vi "Wheel_Control_POS.vi"(9 "CW is Up":bool=TRUE, 10 "AIDeviceRef":T1={"DevStatus"={"status"=FALSE, "code"=0, "source"=""}, "Analog Channel"=enum."AI 1"}, 11 "Wheel DevRef In":T3) -> ()   [LabVIEW 2015, in "Wheel.lvlib"]
doc: "Help by FRC 836 - The RoboBees\n\nThis VI sets the shooter wheel postion using a PID control VI with parameters set by\nthe tbh (Take Back Half) control VI."
uses:
  <userlib>/836-Library/Motion_Control/Shooter_Wheel/Wheel.lvlib
  <userlib>/836-Library/Motion_Control/Shooter_Wheel/WheelControl.ctl
  <userlib>/836-Library/Motion_Control/Shooter_Wheel/Config.ctl
  <userlib>/836-Library/Motion_Control/Shooter_Wheel/Data.ctl
  <vilib>/Rock Robotics/WPI/MotorControl/WPI_MotorControlDeviceRef.ctl
  <vilib>/Rock Robotics/WPI/MotorControl/WPI_MotorControlType.ctl
  <vilib>/Rock Robotics/SystemInterfaces/DIO/FPGA_DIOPWMChannel.ctl
  <vilib>/Rock Robotics/WPI/PWM/WPI_PWMDeadband.ctl
  <vilib>/Rock Robotics/WPI/CAN/Jaguar/SubVIs/WPI_CANJaguar_ControlMode.ctl
  <vilib>/Rock Robotics/WPI/CAN/TalonSRX/WPI_CANTalonSRX_APIControlMode.ctl
  <vilib>/Rock Robotics/WPI/AnalogChannel/WPI_AnalogChannelDevRef.ctl
  <vilib>/Rock Robotics/SystemInterfaces/AI/FPGA_AIChannel.ctl
  <vilib>/Platform/TimedLoop/XDataNode/timing_clust.ctl
  <vilib>/Platform/TimedLoop/XDataNode/nitl_modes.ctl
  <vilib>/Platform/TimedLoop/XDataNode/wakeup.ctl
  <vilib>/addons/control/pid/pid.llb/PID (DBL).vi
  <vilib>/platform/TimedLoop/XDataNode/XDataNode.xnode
  <vilib>/Platform/TimedLoop/XDataNode/XDNodeRunTimeDep.lvlib
  <vilib>/addons/control/pid/NI_PID_pid.lvlib
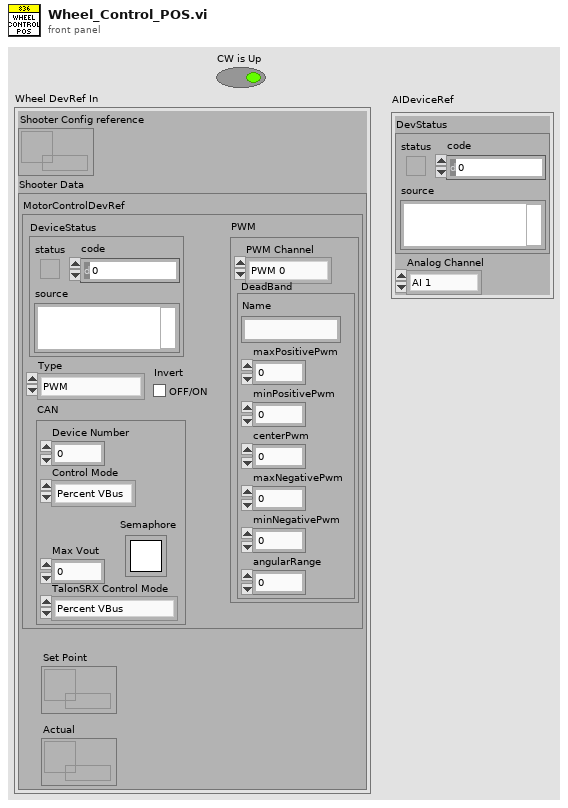
[diagram p1: front panel]
types:
  T1 = typedef "WPI_AnalogChannelDevRef.ctl" = cluster{"DevStatus":errorcluster, "Analog Channel":T2}
  T2 = typedef "FPGA_AIChannel.ctl" = enum8{"AI 0", "AI 1", "AI 2", "AI 3", "AI MXP 0", "AI MXP 1", "AI MXP 2", "AI MXP 3", "Invalid"}
  T3 = typedef "Wheel.lvlib/WheelControl.ctl" = cluster{"Shooter Config reference":refnum<data-value>, "Shooter Data":T4}
  T4 = typedef "Wheel.lvlib/Data.ctl" = cluster{"MotorControlDevRef":T5, "Set Point":refnum<k33>, "Actual":refnum<k33>}
  T5 = typedef "WPI_MotorControlDeviceRef.ctl" = cluster{"DeviceStatus":errorcluster, "Type":T6, "PWM":cluster{"PWM Channel":T7, "DeadBand":T8}, "CAN":cluster{"Device Number":u8, "Control Mode":T9, "Semaphore":T10, "Max Vout":dbl, "TalonSRX Control Mode":T11}, "Invert":bool}
  T6 = typedef "WPI_MotorControlType.ctl" = enum16{"PWM", "CAN", "CANTalonSRX"}
  T7 = typedef "FPGA_DIOPWMChannel.ctl" = enum8{"PWM 0", "PWM 1", "PWM 2", "PWM 3", "PWM 4", "PWM 5", "PWM 6", "PWM 7", "PWM 8", "PWM 9", "PWM MXP 0", "PWM MXP 1", "PWM MXP 2", "PWM MXP 3", "PWM MXP 4", "PWM MXP 5", "PWM MXP 6", "PWM MXP 7", "PWM MXP 8", "PWM MXP 9", "Invalid"}
  T8 = typedef "WPI_PWMDeadband.ctl" = cluster{"Name":string, "maxPositivePwm":i32, "minPositivePwm":i32, "centerPwm":i32, "maxNegativePwm":i32, "minNegativePwm":i32, "angularRange":u16}
  T9 = typedef "WPI_CANJaguar_ControlMode.ctl" = enum8{"Percent VBus", "Current", "Speed", "Position", "Voltage"}
  T10 = typedef "Semaphore RefNum" = refnum<k1>
  T11 = typedef "WPI_CANTalonSRX_APIControlMode.ctl" = enum8{"Percent VBus", "Speed", "Position", "Slave", "Unchanged / Invalid", "Voltage Compensation", "Current", "Motion Profile"}
  T12 = typedef "XDNodeRunTimeDep.lvlib/timing_clust.ctl" = cluster{"Expected End [f-1]":u64, "Actual End [f-1]":u64, "Finished Late? [f-1]":bool, "Expected End [i-1]":u64, "Actual End [i-1]":u64, "Finished Late? [i-1]":bool, "Expected Start [i]":u64, "Actual Start [i]":u64, "Expected Start [f]":u64, "Actual Start [f]":u64, "Source Name":string, "Structure Name":string, "Period":i64, "Deadline":i64, "Offset":i64, "Start":i64, "Priority":i32, "Timeout":i32, "Mode":T13, "Wakeup Reason":T14, "Error":errorcluster, "Source Type":string, "Secondary Source Type":string, "Global End Time":u64, "Global Start Time":u64, "Frame Duration":u64, "Iteration Duration":u64, "Assigned CPU":i32, "I/O Scan Engine Mode":u32}
  T13 = typedef "XDNodeRunTimeDep.lvlib/nitl_modes.ctl" = enum32{"No Change", "Process missed periods, maintain original phase", "Discard missed periods, maintain original phase", "Process missed periods, ignore original phase", "Discard missed periods, ignore original phase"}
  T14 = typedef "XDNodeRunTimeDep.lvlib/wakeup.ctl" = enum32{"Normal", "Aborted", "Asynchronous wakeup", "Timing source error", "Timed loop error", "Timeout"}
  T15 = typedef "Wheel.lvlib/Config.ctl" = cluster{"Period (ms)":i64, "TBH Gain":dbl, "Priority":i32, "PID gains":cluster{"proportional gain (Kc)":dbl, "integral time (Ti, min)":dbl, "derivative time (Td, min)":dbl}, "Stable (sec)":dbl, "Range":dbl}
  T16 = cluster{"proportional gain (Kc)":dbl, "integral time (Ti, min)":dbl, "derivative time (Td, min)":dbl}
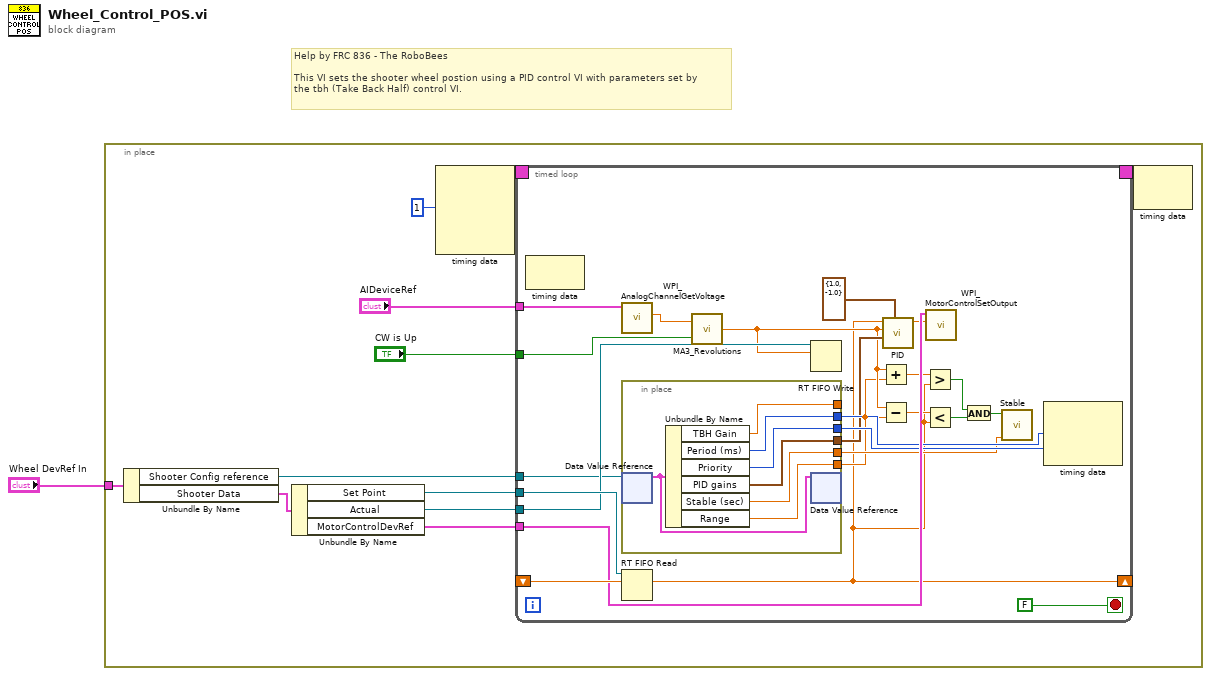
[diagram p0: block diagram]
diagram:
  # "Help by FRC 836 - The RoboBees\n\nThis VI sets the shooter wheel postion using a PID control VI with parameters set by\nthe tbh (Take Back Half) control VI."
  n1 = in-place {
    in-place-border: "Wheel DevRef In" -> [w4]
    n2 = Unbundle By Name(w4) -> ("Shooter Config reference"=w5:refnum<data-value>, "Shooter Data"=w6:T4)
    n3 = Unbundle By Name(w6) -> ("Set Point"=w7:refnum<k33>, "Actual"=w8:refnum<k33>, "MotorControlDevRef"=w10:T5)
    n4 = node-c288(i64 1 ("Period")) -> (w12:T12)  [unwired: 3 in]
    n5 = timed-loop {
      timing: w12 -> [_]
      timing-out: [_] -> w11
      tunnel: w7 -> [w34]
      tunnel: w8 -> [w33]
      shift-right: [w13] -> _
      shift-left: _ -> [w32]
      tunnel: w10 -> [w31]
      tunnel: w5 -> [w30]
      tunnel: "CW is Up" -> [w26]
      tunnel: "AIDeviceRef" -> [w25]
      stop <- FALSE stop-if-true
      n6 = node-c288() -> ()  [unwired: 1 in, 1 out]
      n7 = call <vilib>:"WPI_AnalogChannelGetVoltage.vi"("AIDeviceRef"=w25) -> ("Voltage"=w27:dbl)  [unwired: 8 in, 2 out]
      n8 = in-place {
        in-place-border: [w42] -> _
        in-place-border: [w41] -> w29
        in-place-border: [w40] -> w28
        in-place-border: [w38] -> w23
        in-place-border: [w37] -> w22
        in-place-border: [w36] -> w19
        n9 = in-place-dvr #1(w30) -> (w39:T15)  [unwired: 1 out]
        n10 = Unbundle By Name(w39) -> ("TBH Gain"=w42:dbl, "Period (ms)"=w41:i64, "Priority"=w40:i32, "PID gains"=w38:T16, "Stable (sec)"=w37:dbl, "Range"=w36:dbl)
        n11 = in-place-dvr #1(w39) -> ()  [unwired: 2 out]
      }
      n12 = RT FIFO Read(0:w34, 1:w32) -> (9:w13:dbl)  [unwired: 2 in, 4 out]
      n13 = call <userlib>:"MA3_Revolutions.vi"("CW is Up"=w26, "V in"=w27) -> ("Revs"=w20:dbl)
      n14 = RT FIFO Write(0:w33, 1:w20) -> ()  [unwired: 3 in, 4 out]
      n15 = Add(x=w20, y=w19) -> (x+y=w18:dbl)
      n16 = Subtract(x=w20, y=w19) -> (x-y=w17:dbl)
      n17 = call-poly <vilib>:"PID.vi"("output range"=cluster{"output high":dbl, "output low":dbl} {"output high"=1.0, "output low"=-1.0}, "PID gains"=w23, "process variable"=w20, "setpoint"=w13) -> ("output"=w24:dbl)  [unwired: 6 in, 1 out]
      n18 = Greater?(x=w18, y=w13) -> (0:w16:bool)
      n19 = Less?(x=w17, y=w13) -> (x < y?=w15:bool)
      n20 = call <vilib>:"WPI_MotorControlSetOutput.vi"("Output"=w24, "MotorControlDevRef"=w31) -> ()  [unwired: 7 in, 3 out]
      n21 = And(x=w16, y=w15) -> (x .and. y?=w14:bool)
      n22 = call <userlib>:"Stable.vi"("Eval Period (sec)"=w22, "Signal Input"=w14) -> ()  [unwired: 9 in, 1 out]
      n23 = node-c288(w29, w28) -> ()  [unwired: 1 in, 1 out]
    }
    n24 = node-c288(w11) -> ()  [unwired: 1 out]
  }
